vi "macro_Field_Display_Constant.vi"() -> ()   [LabVIEW 2019, in "Trajectory_Library.lvlib"]
doc: "This WebSockets API example VI acts as a server for an incoming websockets connection. Receives/sends string data to the connected client."
uses:
  TypeDef/FieldDisp_ElementPicture.ctl
  TypeDef/POSE2D.ctl
  TypeDef/TRANSLATION2D.ctl
  TypeDef/ROTATION2D.ctl
  Trajectory_Library.lvlib
panel:
  in  "Robot Pose SI":T1={"TRANSLATION"={"X"=1.0, "Y"=1.0}, "ROTATION"={"VALUE"=0.0, "COS"=1.0, "SIN"=0.0}} {"ROTATION"."SIN" format="%13.4f"; "ROTATION"."COS" format="%13.4f"; "ROTATION"."VALUE" format="%13.4f"; "TRANSLATION"."Y" format="%14.3f"; "TRANSLATION"."X" format="%14.3f"}
  out "ROBOT":T4
  out "Field Picture":picture
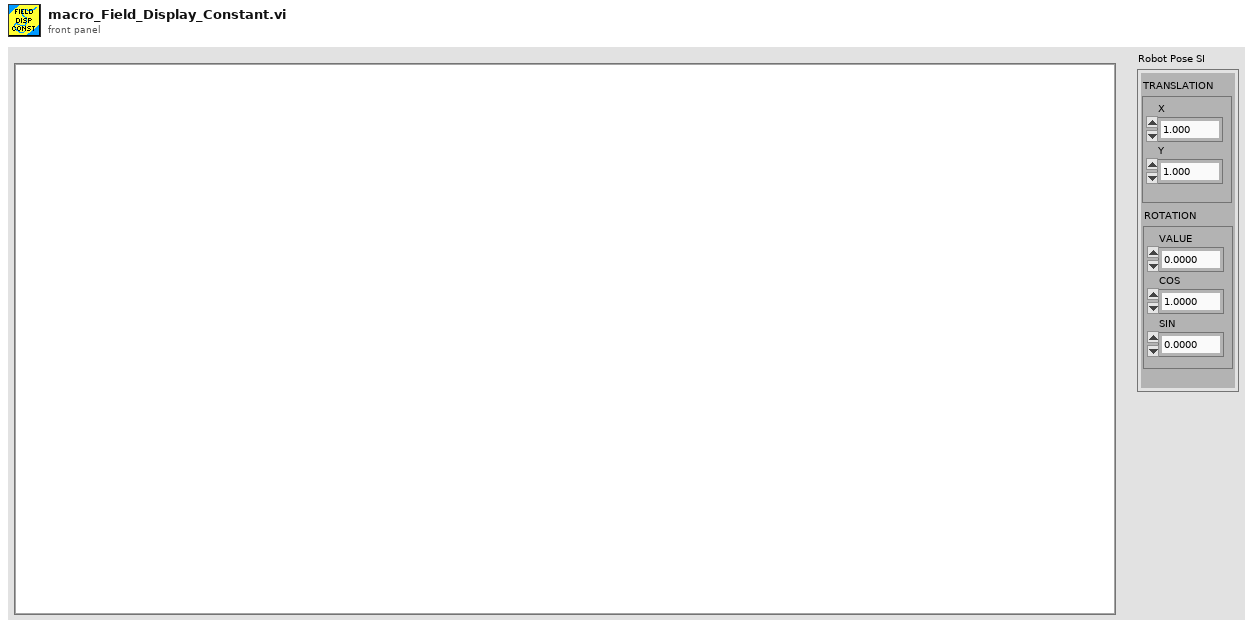
[diagram p1: front panel]
types:
  T1 = typedef "Trajectory_Library.lvlib/POSE2D.ctl" = cluster{"TRANSLATION":T2, "ROTATION":T3}
  T2 = typedef "Trajectory_Library.lvlib/TRANSLATION2D.ctl" = cluster{"X":dbl, "Y":dbl}
  T3 = typedef "Trajectory_Library.lvlib/ROTATION2D.ctl" = cluster{"VALUE":dbl, "COS":dbl, "SIN":dbl}
  T4 = typedef "Trajectory_Library.lvlib/FieldDisp_ElementPicture.ctl" = picture
  T5 = typedef "Trajectory_Library.lvlib/FieldDisp_FieldElement.ctl" = cluster{"ONE-8-bit pixmap":u8[][], "Two-Array":cdb[][], "Three-Numeric":i32, "Four-Numeric":i32, "Five-Numeric":cdb, "Six-colors":u32[], "Seven-new element/subarray":u32, "Left Poxel":dbl, "Top Pixel":dbl, "Width Pix/Ft":dbl, "Height Pix/Ft":dbl, "Element Picture Ref":refnum<vi>}
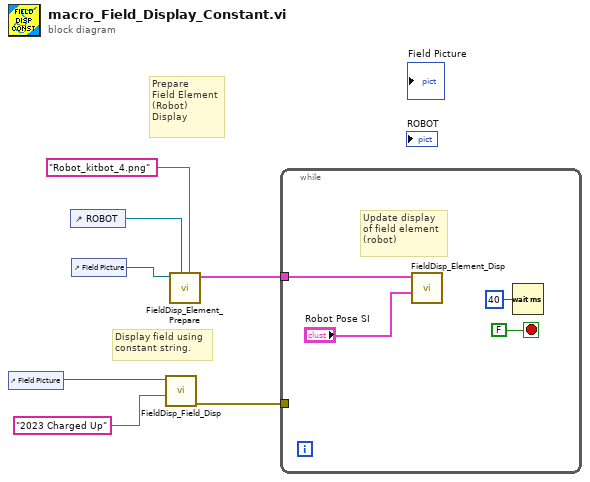
[diagram p0: block diagram]
diagram:
  # "Display field using\nconstant string."
  # "Prepare\nField Element\n(Robot)\nDisplay"
  n1 = control-ref of="Field Picture"() -> (w3:refnum<vi>)
  n2 = control-ref of="ROBOT"() -> (w6:refnum<vi>)
  n3 = control-ref of="Field Picture"() -> (w7:refnum<vi>)
  n4 = call "FieldDisp_Field_Disp.vi"("Field Selector"="2023 Charged Up", "Picture in"=w3) -> ("error out"=w1:errorcluster)  [unwired: 9 in]
  n5 = call "FieldDisp_Element_Prepare.vi"("Element File Name"="Robot_kitbot_4.png" ("Picture FIle Name"), "Element Picture Ref"=w6, "Field Picture Ref"=w7) -> ("Field Element Info"=w4:T5)  [unwired: 7 in, 1 out]
  n6 = while {
    tunnel: w4 -> [w9]
    tunnel: w1 -> [_]
    stop <- FALSE stop-if-true
    # "Update display\nof field element\n(robot)"
    n7 = call "FieldDisp_Element_Disp.vi"("Element Pose"="Robot Pose SI", "Element Info"=w9) -> ()  [unwired: 10 in]
    n8 = Wait (ms)(milliseconds to wait=u32 40) -> ()  [unwired: 1 out]
  }
